vi "Lab Panel V4.83.vi"() -> ()   [LabVIEW 2013] (continued)
                        n580 = case shown="\"CYCLE TEST\"" w902 {
                          tunnel: w900 -> [_ _ w909]
                          tunnel: w899 -> [w907 w908 _]
                          tunnel: [w907 w908 w909] -> w898
                          frame "CHART TEST", Default {
                          }
                          frame "CYCLE TEST" {
                          }
                          frame "T-RISE TEST" {
                          }
                        }
                        n581 = local read "TDMS LAB02-2"() -> (w906:refnum<k34>)
                        n582 = Build Array("STOPPED") -> (w903:string[])
                        n583 = Build Array(w898) -> (w897:dbl[])
                        n584 = TDMS Write(0:w906, 5:"TEST RESULT", 7:w903, 9:w897) -> (4:w895:refnum<k34>, 15:w896:errorcluster)  [unwired: 2 in, 2 out]
                        n585 = TDMS Close(8:w896, 11:w895) -> (0:w894:errorcluster)  [unwired: 1 out]
                      }
                      frame #1 {
                        n586 = local read "DISP LAB02-2"() -> (w913:T4)
                        n587 = stacked-sequence {
                          tunnel: "LAB02-2" -> [w915 w917]
                          frame #0 {
                            n588 = call "sub vi - defrag tdms v1.vi"("panel id"=w915) -> ("error out"=w914:errorcluster)  [unwired: 10 in]
                            n589 = local write "data file error"(w914) -> ()
                          }
                          frame #1 {
                            n590 = call "Save data file to network drive v1.vi"("panel id"=w917) -> ("network file save error"=w916:errorcluster)  [unwired: 9 in, 1 out]
                            n591 = local write "RESULT LAB02-2"(FALSE) -> ()
                            n592 = local write "data file error"(w916) -> ()
                          }
                        }
                        n593 = Bundle(cluster=w913, "STATUS"="STOP") -> (w911:T4)  [unwired: 2 in]
                        n594 = local write "DISP LAB02-2"(w911) -> ()
                      }
                    }
                  }
                  frame True {
                    # "start new test and create test file"
                    n595 = stacked-sequence {
                      seq-local: [w925 _ _ _ _] -> [_ w950 _ _ _]
                      tunnel: w924 -> [w930 _ _ _ _]
                      tunnel: w923 -> [w927 _ _ _ _]
                      tunnel: w922 -> [w940 _ _ _ _]
                      tunnel: w921 -> [w933 _ _ _ _]
                      tunnel: w920 -> [w928 _ _ _ _]
                      tunnel: [_ w944 _ _ _] -> w919
                      frame #0 {
                        w926 = "\\"
                        n596 = local read "SET LAB02-2"() -> (w935:T5)
                        n597 = case shown="\"CYCLE TEST\"" w940 {
                          tunnel: ["L02-2-CHART TEST-" "L02-2-CYCLE TEST-" "L02-2-T-RISE TEST-"] -> w936
                          frame "CHART TEST", Default {
                          }
                          frame "CYCLE TEST" {
                          }
                          frame "T-RISE TEST" {
                          }
                        }
                        n598 = Unbundle(w935) -> ("DESCRIPTION"=w934:string)  [unwired: 4 out]
                        n599 = Concatenate Strings(w930, "\\", w928, w926, w927, w926) -> (w937:string)
                        n600 = String To Path(string=w937) -> (path=w939:path)
                        n601 = Concatenate Strings(w937, w936, w934, "-", w933, ".tdms") -> (w925:string)
                        n602 = Create Folder(path (use dialog)=w939) -> (error out=w938:errorcluster)  [unwired: 2 in, 2 out]
                        n603 = global write "Global 1.vi" "LAB02-2 FILE"(w925) -> ()
                        n604 = call <vilib>:"Clear Errors.vi"("error in (no error)"=w938) -> ()  [unwired: 6 in, 1 out]
                      }
                      frame #1 {
                        n605 = String To Path(string=w950) -> (path=w945:path)
                        n606 = TDMS Open(5:FALSE, 6:FALSE, 10:T18."create or replace" ("operation (0:open)"), 11:w945) -> (0:w944:errorcluster, 3:→"TDMS LAB02-2":refnum<k34>)  [unwired: 3 in]
                      }
                      frame #2 {
                        n607 = local read "SET LAB02-2"() -> (w956:T5)
                        n608 = local read "TDMS LAB02-2"() -> (w967:refnum<k34>)
                        n609 = Build Array("Testers Name", "Description", "Set Test Cycles", "T-Rise minutes", "T-Rise Deg C") -> (w957:string[])
                        n610 = Unbundle(w956) -> ("NAME"=w955:string, "DESCRIPTION"=w954:string, "CYCLES"=w953:dbl, "T-RISE mins"=w952:dbl, "T-RISE deg C"=w951:dbl)
                        n611 = Number To Decimal String(number=w953) -> (decimal integer string=w966:string)  [unwired: 1 in]
                        n612 = Number To Decimal String(number=w952) -> (decimal integer string=w965:string)  [unwired: 1 in]
                        n613 = Number To Decimal String(number=w951) -> (decimal integer string=w964:string)  [unwired: 1 in]
                        n614 = Build Array(w955, w954, w966, w965, w964) -> (w963:string[])
                        n615 = TDMS Set Properties(5:w963, 7:w957, 11:w967) -> ()  [unwired: 3 in, 4 out]
                      }
                      frame #3 {
                        w969 = 0.0
                        n616 = local read "DISP LAB02-2"() -> (w971:T4)
                        n617 = Bundle(cluster=w971, "CYCLE"=w969, "MINS"=w969, "STATUS"="RUN") -> (w970:T4)
                        n618 = local write "DISP LAB02-2"(w970) -> ()
                      }
                      frame #4 {
                        n619 = local read "SIG LAB02-2"() -> (w974:T2)
                        n620 = local read "TEMP START LAB02-2"() -> (w976:cluster{"TL":dbl, "TN":dbl})
                        n621 = Unbundle(w974) -> ("Tmp Live"=w973:dbl, "Tmp Neut"=w972:dbl)  [unwired: 3 out]
                        n622 = Bundle(cluster=w976, "TL"=w973, "TN"=w972) -> (w975:cluster{"TL":dbl, "TN":dbl})
                        n623 = local write "TEMP START LAB02-2"(w975) -> ()
                      }
                    }
                  }
                }
              }
              event "RUN LAB03-1": Value Change {
                n624 = event-data() -> ("NewVal"=w977:bool)  [unwired: 1 in, 5 out]
                n625 = local write "run lab03-1"(w977) -> ()
                n626 = case shown="True" w977 {
                  tunnel: w983 -> [_ w1016]
                  tunnel: w982 -> [_ w1015]
                  tunnel: w980 -> [w985 w1014]
                  tunnel: w981 -> [_ w1013]
                  tunnel: w979 -> [_ w1012]
                  tunnel: [w984 w1011] -> w978
                  frame False {
                    # "stop test"
                    n627 = stacked-sequence {
                      tunnel: w985 -> [w994 _]
                      tunnel: [w986 _] -> w984
                      frame #0 {
                        n628 = local read "DISP LAB03-1"() -> (w993:T4)
                        n629 = Unbundle(w993) -> ("CYCLE"=w991:dbl, "MINS"=w992:dbl)  [unwired: 1 out]
                        n630 = case shown="\"CYCLE TEST\"" w994 {
                          tunnel: w992 -> [_ _ w1001]
                          tunnel: w991 -> [w999 w1000 _]
                          tunnel: [w999 w1000 w1001] -> w990
                          frame "CHART TEST", Default {
                          }
                          frame "CYCLE TEST" {
                          }
                          frame "T-RISE TEST" {
                          }
                        }
                        n631 = local read "TDMS LAB03-1"() -> (w998:refnum<k34>)
                        n632 = Build Array("STOPPED") -> (w995:string[])
                        n633 = Build Array(w990) -> (w989:dbl[])
                        n634 = TDMS Write(0:w998, 5:"TEST RESULT", 7:w995, 9:w989) -> (4:w987:refnum<k34>, 15:w988:errorcluster)  [unwired: 2 in, 2 out]
                        n635 = TDMS Close(8:w988, 11:w987) -> (0:w986:errorcluster)  [unwired: 1 out]
                      }
                      frame #1 {
                        n636 = local read "DISP LAB03-1"() -> (w1005:T4)
                        n637 = stacked-sequence {
                          tunnel: "LAB03-1" -> [w1007 w1009]
                          frame #0 {
                            n638 = call "sub vi - defrag tdms v1.vi"("panel id"=w1007) -> ("error out"=w1006:errorcluster)  [unwired: 10 in]
                            n639 = local write "data file error"(w1006) -> ()
                          }
                          frame #1 {
                            n640 = call "Save data file to network drive v1.vi"("panel id"=w1009) -> ("network file save error"=w1008:errorcluster)  [unwired: 9 in, 1 out]
                            n641 = local write "RESULT LAB03-1"(FALSE) -> ()
                            n642 = local write "data file error"(w1008) -> ()
                          }
                        }
                        n643 = Bundle(cluster=w1005, "STATUS"="STOP") -> (w1003:T4)  [unwired: 2 in]
                        n644 = local write "DISP LAB03-1"(w1003) -> ()
                      }
                    }
                  }
                  frame True {
                    # "start new test and create test file"
                    n645 = stacked-sequence {
                      seq-local: [w1017 _ _ _ _] -> [_ w1042 _ _ _]
                      tunnel: w1016 -> [w1022 _ _ _ _]
                      tunnel: w1015 -> [w1019 _ _ _ _]
                      tunnel: w1014 -> [w1032 _ _ _ _]
                      tunnel: w1013 -> [w1025 _ _ _ _]
                      tunnel: w1012 -> [w1020 _ _ _ _]
                      tunnel: [_ w1036 _ _ _] -> w1011
                      frame #0 {
                        w1018 = "\\"
                        n646 = local read "SET LAB03-1"() -> (w1027:T5)
                        n647 = case shown="\"T-RISE TEST\"" w1032 {
                          tunnel: ["L03-1-CHART TEST-" "L03-1-CYCLE TEST-" "L03-1-T-RISE TEST-"] -> w1028
                          frame "CHART TEST", Default {
                          }
                          frame "CYCLE TEST" {
                          }
                          frame "T-RISE TEST" {
                          }
                        }
                        n648 = Unbundle(w1027) -> ("DESCRIPTION"=w1026:string)  [unwired: 4 out]
                        n649 = Concatenate Strings(w1022, "\\", w1020, w1018, w1019, w1018) -> (w1029:string)
                        n650 = String To Path(string=w1029) -> (path=w1031:path)
                        n651 = Concatenate Strings(w1029, w1028, w1026, "-", w1025, ".tdms") -> (w1017:string)
                        n652 = Create Folder(path (use dialog)=w1031) -> (error out=w1030:errorcluster)  [unwired: 2 in, 2 out]
                        n653 = global write "Global 1.vi" "LAB03-1 FILE"(w1017) -> ()
                        n654 = call <vilib>:"Clear Errors.vi"("error in (no error)"=w1030) -> ()  [unwired: 6 in, 1 out]
                      }
                      frame #1 {
                        n655 = String To Path(string=w1042) -> (path=w1037:path)
                        n656 = TDMS Open(5:FALSE, 6:FALSE, 10:T18."create or replace" ("operation (0:open)"), 11:w1037) -> (0:w1036:errorcluster, 3:→"TDMS LAB03-1":refnum<k34>)  [unwired: 3 in]
                      }
                      frame #2 {
                        n657 = local read "SET LAB03-1"() -> (w1048:T5)
                        n658 = local read "TDMS LAB03-1"() -> (w1059:refnum<k34>)
                        n659 = Build Array("Testers Name", "Description", "Set Test Cycles", "T-Rise minutes", "T-Rise Deg C") -> (w1049:string[])
                        n660 = Unbundle(w1048) -> ("NAME"=w1047:string, "DESCRIPTION"=w1046:string, "CYCLES"=w1045:dbl, "T-RISE mins"=w1044:dbl, "T-RISE deg C"=w1043:dbl)
                        n661 = Number To Decimal String(number=w1045) -> (decimal integer string=w1058:string)  [unwired: 1 in]
                        n662 = Number To Decimal String(number=w1044) -> (decimal integer string=w1057:string)  [unwired: 1 in]
                        n663 = Number To Decimal String(number=w1043) -> (decimal integer string=w1056:string)  [unwired: 1 in]
                        n664 = Build Array(w1047, w1046, w1058, w1057, w1056) -> (w1055:string[])
                        n665 = TDMS Set Properties(5:w1055, 7:w1049, 11:w1059) -> ()  [unwired: 3 in, 4 out]
                      }
                      frame #3 {
                        w1061 = 0.0
                        n666 = local read "DISP LAB03-1"() -> (w1063:T4)
                        n667 = Bundle(cluster=w1063, "CYCLE"=w1061, "MINS"=w1061, "STATUS"="RUN") -> (w1062:T4)
                        n668 = local write "DISP LAB03-1"(w1062) -> ()
                      }
                      frame #4 {
                        n669 = local read "SIG LAB03-1"() -> (w1066:T2)
                        n670 = local read "TEMP START LAB03-1"() -> (w1068:cluster{"TL":dbl, "TN":dbl})
                        n671 = Unbundle(w1066) -> ("Tmp Live"=w1065:dbl, "Tmp Neut"=w1064:dbl)  [unwired: 3 out]
                        n672 = Bundle(cluster=w1068, "TL"=w1065, "TN"=w1064) -> (w1067:cluster{"TL":dbl, "TN":dbl})
                        n673 = local write "TEMP START LAB03-1"(w1067) -> ()
                      }
                    }
                  }
                }
              }
              event "RUN LAB03-2": Value Change {
                n674 = event-data() -> ("NewVal"=w1069:bool)  [unwired: 1 in, 5 out]
                n675 = local write "run lab03-2"(w1069) -> ()
                n676 = case shown="True" w1069 {
                  tunnel: w1075 -> [_ w1108]
                  tunnel: w1074 -> [_ w1107]
                  tunnel: w1072 -> [w1077 w1106]
                  tunnel: w1073 -> [_ w1105]
                  tunnel: w1071 -> [_ w1104]
                  tunnel: [w1076 w1103] -> w1070
                  frame False {
                    # "stop test"
                    n677 = stacked-sequence {
                      tunnel: w1077 -> [w1086 _]
                      tunnel: [w1078 _] -> w1076
                      frame #0 {
                        n678 = local read "DISP LAB03-2"() -> (w1085:T4)
                        n679 = Unbundle(w1085) -> ("CYCLE"=w1083:dbl, "MINS"=w1084:dbl)  [unwired: 1 out]
                        n680 = case shown="\"CYCLE TEST\"" w1086 {
                          tunnel: w1084 -> [_ _ w1093]
                          tunnel: w1083 -> [w1091 w1092 _]
                          tunnel: [w1091 w1092 w1093] -> w1082
                          frame "CHART TEST", Default {
                          }
                          frame "CYCLE TEST" {
                          }
                          frame "T-RISE TEST" {
                          }
                        }
                        n681 = local read "TDMS LAB03-2"() -> (w1090:refnum<k34>)
                        n682 = Build Array("STOPPED") -> (w1087:string[])
                        n683 = Build Array(w1082) -> (w1081:dbl[])
                        n684 = TDMS Write(0:w1090, 5:"TEST RESULT", 7:w1087, 9:w1081) -> (4:w1079:refnum<k34>, 15:w1080:errorcluster)  [unwired: 2 in, 2 out]
                        n685 = TDMS Close(8:w1080, 11:w1079) -> (0:w1078:errorcluster)  [unwired: 1 out]
                      }
                      frame #1 {
                        n686 = local read "DISP LAB03-2"() -> (w1097:T4)
                        n687 = stacked-sequence {
                          tunnel: "LAB03-2" -> [w1099 w1101]
                          frame #0 {
                            n688 = call "sub vi - defrag tdms v1.vi"("panel id"=w1099) -> ("error out"=w1098:errorcluster)  [unwired: 10 in]
                            n689 = local write "data file error"(w1098) -> ()
                          }
                          frame #1 {
                            n690 = call "Save data file to network drive v1.vi"("panel id"=w1101) -> ("network file save error"=w1100:errorcluster)  [unwired: 9 in, 1 out]
                            n691 = local write "RESULT LAB03-2"(FALSE) -> ()
                            n692 = local write "data file error"(w1100) -> ()
                          }
                        }
                        n693 = Bundle(cluster=w1097, "STATUS"="STOP") -> (w1095:T4)  [unwired: 2 in]
                        n694 = local write "DISP LAB03-2"(w1095) -> ()
                      }
                    }
                  }
                  frame True {
                    # "start new test and create test file"
                    n695 = stacked-sequence {
                      seq-local: [w1109 _ _ _ _] -> [_ w1134 _ _ _]
                      tunnel: w1108 -> [w1114 _ _ _ _]
                      tunnel: w1107 -> [w1111 _ _ _ _]
                      tunnel: w1106 -> [w1124 _ _ _ _]
                      tunnel: w1105 -> [w1117 _ _ _ _]
                      tunnel: w1104 -> [w1112 _ _ _ _]
                      tunnel: [_ w1128 _ _ _] -> w1103
                      frame #0 {
                        w1110 = "\\"
                        n696 = local read "SET LAB03-2"() -> (w1119:T5)
                        n697 = case shown="\"T-RISE TEST\"" w1124 {
                          tunnel: ["L03-2-CHART TEST-" "L03-2-CYCLE TEST-" "L03-2-T-RISE TEST-"] -> w1120
                          frame "CHART TEST", Default {
                          }
                          frame "CYCLE TEST" {
                          }
                          frame "T-RISE TEST" {
                          }
                        }
                        n698 = Unbundle(w1119) -> ("DESCRIPTION"=w1118:string)  [unwired: 4 out]
                        n699 = Concatenate Strings(w1114, "\\", w1112, w1110, w1111, w1110) -> (w1121:string)
                        n700 = String To Path(string=w1121) -> (path=w1123:path)
                        n701 = Concatenate Strings(w1121, w1120, w1118, "-", w1117, ".tdms") -> (w1109:string)
                        n702 = Create Folder(path (use dialog)=w1123) -> (error out=w1122:errorcluster)  [unwired: 2 in, 2 out]
                        n703 = global write "Global 1.vi" "LAB03-2 FILE"(w1109) -> ()
                        n704 = call <vilib>:"Clear Errors.vi"("error in (no error)"=w1122) -> ()  [unwired: 6 in, 1 out]
                      }
                      frame #1 {
                        n705 = String To Path(string=w1134) -> (path=w1129:path)
                        n706 = TDMS Open(5:FALSE, 6:FALSE, 10:T18."create or replace" ("operation (0:open)"), 11:w1129) -> (0:w1128:errorcluster, 3:→"TDMS LAB03-2":refnum<k34>)  [unwired: 3 in]
                      }
                      frame #2 {
                        n707 = local read "SET LAB03-2"() -> (w1140:T5)
                        n708 = local read "TDMS LAB03-2"() -> (w1151:refnum<k34>)
                        n709 = Build Array("Testers Name", "Description", "Set Test Cycles", "T-Rise minutes", "T-Rise Deg C") -> (w1141:string[])
                        n710 = Unbundle(w1140) -> ("NAME"=w1139:string, "DESCRIPTION"=w1138:string, "CYCLES"=w1137:dbl, "T-RISE mins"=w1136:dbl, "T-RISE deg C"=w1135:dbl)
                        n711 = Number To Decimal String(number=w1137) -> (decimal integer string=w1150:string)  [unwired: 1 in]
                        n712 = Number To Decimal String(number=w1136) -> (decimal integer string=w1149:string)  [unwired: 1 in]
                        n713 = Number To Decimal String(number=w1135) -> (decimal integer string=w1148:string)  [unwired: 1 in]
                        n714 = Build Array(w1139, w1138, w1150, w1149, w1148) -> (w1147:string[])
                        n715 = TDMS Set Properties(5:w1147, 7:w1141, 11:w1151) -> ()  [unwired: 3 in, 4 out]
                      }
                      frame #3 {
                        w1153 = 0.0
                        n716 = local read "DISP LAB03-2"() -> (w1155:T4)
                        n717 = Bundle(cluster=w1155, "CYCLE"=w1153, "MINS"=w1153, "STATUS"="RUN") -> (w1154:T4)
                        n718 = local write "DISP LAB03-2"(w1154) -> ()
                      }
                      frame #4 {
                        n719 = local read "SIG LAB03-2"() -> (w1158:T2)
                        n720 = local read "TEMP START LAB03-2"() -> (w1160:cluster{"TL":dbl, "TN":dbl})
                        n721 = Unbundle(w1158) -> ("Tmp Live"=w1157:dbl, "Tmp Neut"=w1156:dbl)  [unwired: 3 out]
                        n722 = Bundle(cluster=w1160, "TL"=w1157, "TN"=w1156) -> (w1159:cluster{"TL":dbl, "TN":dbl})
                        n723 = local write "TEMP START LAB03-2"(w1159) -> ()
                      }
                    }
                  }
                }
              }
              event "RUN LAB04-1": Value Change {
                n724 = event-data() -> ("NewVal"=w1161:bool)  [unwired: 1 in, 5 out]
                n725 = local write "run lab04-1"(w1161) -> ()
                n726 = case shown="True" w1161 {
                  tunnel: w1167 -> [_ w1200]
                  tunnel: w1166 -> [_ w1199]
                  tunnel: w1164 -> [w1169 w1198]
                  tunnel: w1165 -> [_ w1197]
                  tunnel: w1163 -> [_ w1196]
                  tunnel: [w1168 w1195] -> w1162
                  frame False {
                    # "stop test"
                    n727 = stacked-sequence {
                      tunnel: w1169 -> [w1178 _]
                      tunnel: [w1170 _] -> w1168
                      frame #0 {
                        n728 = local read "DISP LAB04-1"() -> (w1177:T4)
                        n729 = Unbundle(w1177) -> ("CYCLE"=w1175:dbl, "MINS"=w1176:dbl)  [unwired: 1 out]
                        n730 = case shown="\"CYCLE TEST\"" w1178 {
                          tunnel: w1176 -> [_ _ w1185]
                          tunnel: w1175 -> [w1183 w1184 _]
                          tunnel: [w1183 w1184 w1185] -> w1174
                          frame "CHART TEST", Default {
                          }
                          frame "CYCLE TEST" {
                          }
                          frame "T-RISE TEST" {
                          }
                        }
                        n731 = local read "TDMS LAB04-1"() -> (w1182:refnum<k34>)
                        n732 = Build Array("STOPPED") -> (w1179:string[])
                        n733 = Build Array(w1174) -> (w1173:dbl[])
                        n734 = TDMS Write(0:w1182, 5:"TEST RESULT", 7:w1179, 9:w1173) -> (4:w1171:refnum<k34>, 15:w1172:errorcluster)  [unwired: 2 in, 2 out]
                        n735 = TDMS Close(8:w1172, 11:w1171) -> (0:w1170:errorcluster)  [unwired: 1 out]
                      }
                      frame #1 {
                        n736 = local read "DISP LAB04-1"() -> (w1189:T4)
                        n737 = stacked-sequence {
                          tunnel: "LAB04-1" -> [w1191 w1193]
                          frame #0 {
                            n738 = call "sub vi - defrag tdms v1.vi"("panel id"=w1191) -> ("error out"=w1190:errorcluster)  [unwired: 10 in]
                            n739 = local write "data file error"(w1190) -> ()
                          }
                          frame #1 {
                            n740 = call "Save data file to network drive v1.vi"("panel id"=w1193) -> ("network file save error"=w1192:errorcluster)  [unwired: 9 in, 1 out]
                            n741 = local write "RESULT LAB04-1"(FALSE) -> ()
                            n742 = local write "data file error"(w1192) -> ()
                          }
                        }
                        n743 = Bundle(cluster=w1189, "STATUS"="STOP") -> (w1187:T4)  [unwired: 2 in]
                        n744 = local write "DISP LAB04-1"(w1187) -> ()
                      }
                    }
                  }
                  frame True {
                    # "start new test and create test file"
                    n745 = stacked-sequence {
                      seq-local: [w1201 _ _ _ _] -> [_ w1226 _ _ _]
                      tunnel: w1200 -> [w1206 _ _ _ _]
                      tunnel: w1199 -> [w1202 _ _ _ _]
                      tunnel: w1198 -> [w1216 _ _ _ _]
                      tunnel: w1197 -> [w1209 _ _ _ _]
                      tunnel: w1196 -> [w1204 _ _ _ _]
                      tunnel: [_ w1220 _ _ _] -> w1195
                      frame #0 {
                        w1203 = "\\"
                        n746 = local read "SET LAB04-1"() -> (w1211:T5)
                        n747 = case shown="\"CYCLE TEST\"" w1216 {
                          tunnel: ["L04-1-CHART TEST-" "L04-1-CYCLE TEST-" "L04-1-T-RISE TEST-"] -> w1212
                          frame "CHART TEST", Default {
                          }
                          frame "CYCLE TEST" {
                          }
                          frame "T-RISE TEST" {
                          }
                        }
                        n748 = Unbundle(w1211) -> ("DESCRIPTION"=w1210:string)  [unwired: 4 out]
                        n749 = Concatenate Strings(w1206, "\\", w1204, w1203, w1202, w1203) -> (w1213:string)
                        n750 = String To Path(string=w1213) -> (path=w1215:path)
                        n751 = Concatenate Strings(w1213, w1212, w1210, "-", w1209, ".tdms") -> (w1201:string)
                        n752 = Create Folder(path (use dialog)=w1215) -> (error out=w1214:errorcluster)  [unwired: 2 in, 2 out]
                        n753 = global write "Global 1.vi" "LAB04-1 FILE"(w1201) -> ()
                        n754 = call <vilib>:"Clear Errors.vi"("error in (no error)"=w1214) -> ()  [unwired: 6 in, 1 out]
                      }
                      frame #1 {
                        n755 = String To Path(string=w1226) -> (path=w1221:path)
                        n756 = TDMS Open(5:FALSE, 6:FALSE, 10:T18."create or replace" ("operation (0:open)"), 11:w1221) -> (0:w1220:errorcluster, 3:→"TDMS LAB04-1":refnum<k34>)  [unwired: 3 in]
                      }
                      frame #2 {
                        n757 = local read "SET LAB04-1"() -> (w1232:T5)
                        n758 = local read "TDMS LAB04-1"() -> (w1243:refnum<k34>)
                        n759 = Build Array("Testers Name", "Description", "Set Test Cycles", "T-Rise minutes", "T-Rise Deg C") -> (w1233:string[])
                        n760 = Unbundle(w1232) -> ("NAME"=w1231:string, "DESCRIPTION"=w1230:string, "CYCLES"=w1229:dbl, "T-RISE mins"=w1228:dbl, "T-RISE deg C"=w1227:dbl)
                        n761 = Number To Decimal String(number=w1229) -> (decimal integer string=w1242:string)  [unwired: 1 in]
                        n762 = Number To Decimal String(number=w1228) -> (decimal integer string=w1241:string)  [unwired: 1 in]
                        n763 = Number To Decimal String(number=w1227) -> (decimal integer string=w1240:string)  [unwired: 1 in]
                        n764 = Build Array(w1231, w1230, w1242, w1241, w1240) -> (w1239:string[])
                        n765 = TDMS Set Properties(5:w1239, 7:w1233, 11:w1243) -> ()  [unwired: 3 in, 4 out]
                      }
                      frame #3 {
                        w1245 = 0.0
                        n766 = local read "DISP LAB04-1"() -> (w1247:T4)
                        n767 = Bundle(cluster=w1247, "CYCLE"=w1245, "MINS"=w1245, "STATUS"="RUN") -> (w1246:T4)
                        n768 = local write "DISP LAB04-1"(w1246) -> ()
                      }
                      frame #4 {
                        n769 = local read "SIG LAB04-1"() -> (w1250:T2)
                        n770 = local read "TEMP START LAB04-1"() -> (w1252:cluster{"TL":dbl, "TN":dbl})
                        n771 = Unbundle(w1250) -> ("Tmp Live"=w1249:dbl, "Tmp Neut"=w1248:dbl)  [unwired: 3 out]
                        n772 = Bundle(cluster=w1252, "TL"=w1249, "TN"=w1248) -> (w1251:cluster{"TL":dbl, "TN":dbl})
                        n773 = local write "TEMP START LAB04-1"(w1251) -> ()
                      }
                    }
                  }
                }
              }
              event "RUN LAB04-2": Value Change {
                n774 = event-data() -> ("NewVal"=w1253:bool)  [unwired: 1 in, 5 out]
                n775 = local write "run lab04-2"(w1253) -> ()
                n776 = case shown="True" w1253 {
                  tunnel: w1259 -> [_ w1292]
                  tunnel: w1258 -> [_ w1291]
                  tunnel: w1256 -> [w1261 w1290]
                  tunnel: w1257 -> [_ w1289]
                  tunnel: w1255 -> [_ w1288]
                  tunnel: [w1260 w1287] -> w1254
                  frame False {
                    # "stop test"
                    n777 = stacked-sequence {
                      tunnel: w1261 -> [w1270 _]
                      tunnel: [w1262 _] -> w1260
                      frame #0 {
                        n778 = local read "DISP LAB04-2"() -> (w1269:T4)
                        n779 = Unbundle(w1269) -> ("CYCLE"=w1267:dbl, "MINS"=w1268:dbl)  [unwired: 1 out]
                        n780 = case shown="\"CYCLE TEST\"" w1270 {
                          tunnel: w1268 -> [_ _ w1277]
                          tunnel: w1267 -> [w1275 w1276 _]
                          tunnel: [w1275 w1276 w1277] -> w1266
                          frame "CHART TEST", Default {
                          }
                          frame "CYCLE TEST" {
                          }
                          frame "T-RISE TEST" {
                          }
                        }
                        n781 = local read "TDMS LAB04-2"() -> (w1274:refnum<k34>)
                        n782 = Build Array("STOPPED") -> (w1271:string[])
                        n783 = Build Array(w1266) -> (w1265:dbl[])
                        n784 = TDMS Write(0:w1274, 5:"TEST RESULT", 7:w1271, 9:w1265) -> (4:w1263:refnum<k34>, 15:w1264:errorcluster)  [unwired: 2 in, 2 out]
                        n785 = TDMS Close(8:w1264, 11:w1263) -> (0:w1262:errorcluster)  [unwired: 1 out]
                      }
                      frame #1 {
                        n786 = local read "DISP LAB04-2"() -> (w1281:T4)
                        n787 = stacked-sequence {
                          tunnel: "LAB04-2" -> [w1283 w1285]
                          frame #0 {
                            n788 = call "sub vi - defrag tdms v1.vi"("panel id"=w1283) -> ("error out"=w1282:errorcluster)  [unwired: 10 in]
                            n789 = local write "data file error"(w1282) -> ()
                          }
                          frame #1 {
                            n790 = call "Save data file to network drive v1.vi"("panel id"=w1285) -> ("network file save error"=w1284:errorcluster)  [unwired: 9 in, 1 out]
                            n791 = local write "RESULT LAB04-2"(FALSE) -> ()
                            n792 = local write "data file error"(w1284) -> ()
                          }
                        }
                        n793 = Bundle(cluster=w1281, "STATUS"="STOP") -> (w1279:T4)  [unwired: 2 in]
                        n794 = local write "DISP LAB04-2"(w1279) -> ()
                      }
                    }
                  }
                  frame True {
                    # "start new test and create test file"
                    n795 = stacked-sequence {
                      seq-local: [w1293 _ _ _ _] -> [_ w1318 _ _ _]
                      tunnel: w1292 -> [w1298 _ _ _ _]
                      tunnel: w1291 -> [w1294 _ _ _ _]
                      tunnel: w1290 -> [w1308 _ _ _ _]
                      tunnel: w1289 -> [w1301 _ _ _ _]
                      tunnel: w1288 -> [w1296 _ _ _ _]
                      tunnel: [_ w1312 _ _ _] -> w1287
                      frame #0 {
                        w1295 = "\\"
                        n796 = local read "SET LAB04-2"() -> (w1303:T5)
                        n797 = case shown="\"CHART TEST\", Default" w1308 {
                          tunnel: ["L04-2-CHART TEST-" "L04-2-CYCLE TEST-" "L04-2-T-RISE TEST-"] -> w1304
                          frame "CHART TEST", Default {
                          }
                          frame "CYCLE TEST" {
                          }
                          frame "T-RISE TEST" {
                          }
                        }
                        n798 = Unbundle(w1303) -> ("DESCRIPTION"=w1302:string)  [unwired: 4 out]
                        n799 = Concatenate Strings(w1298, "\\", w1296, w1295, w1294, w1295) -> (w1305:string)
                        n800 = String To Path(string=w1305) -> (path=w1307:path)
                        n801 = Concatenate Strings(w1305, w1304, w1302, "-", w1301, ".tdms") -> (w1293:string)
                        n802 = Create Folder(path (use dialog)=w1307) -> (error out=w1306:errorcluster)  [unwired: 2 in, 2 out]
                        n803 = global write "Global 1.vi" "LAB04-2 FILE"(w1293) -> ()
                        n804 = call <vilib>:"Clear Errors.vi"("error in (no error)"=w1306) -> ()  [unwired: 6 in, 1 out]
                      }
                      frame #1 {
                        n805 = String To Path(string=w1318) -> (path=w1313:path)
                        n806 = TDMS Open(5:FALSE, 6:FALSE, 10:T18."create or replace" ("operation (0:open)"), 11:w1313) -> (0:w1312:errorcluster, 3:→"TDMS LAB04-2":refnum<k34>)  [unwired: 3 in]
                      }
                      frame #2 {
                        n807 = local read "SET LAB04-2"() -> (w1324:T5)
                        n808 = local read "TDMS LAB04-2"() -> (w1335:refnum<k34>)
                        n809 = Build Array("Testers Name", "Description", "Set Test Cycles", "T-Rise minutes", "T-Rise Deg C") -> (w1325:string[])
                        n810 = Unbundle(w1324) -> ("NAME"=w1323:string, "DESCRIPTION"=w1322:string, "CYCLES"=w1321:dbl, "T-RISE mins"=w1320:dbl, "T-RISE deg C"=w1319:dbl)
                        n811 = Number To Decimal String(number=w1321) -> (decimal integer string=w1334:string)  [unwired: 1 in]
                        n812 = Number To Decimal String(number=w1320) -> (decimal integer string=w1333:string)  [unwired: 1 in]
                        n813 = Number To Decimal String(number=w1319) -> (decimal integer string=w1332:string)  [unwired: 1 in]
                        n814 = Build Array(w1323, w1322, w1334, w1333, w1332) -> (w1331:string[])
                        n815 = TDMS Set Properties(5:w1331, 7:w1325, 11:w1335) -> ()  [unwired: 3 in, 4 out]
                      }
                      frame #3 {
                        w1337 = 0.0
                        n816 = local read "DISP LAB04-2"() -> (w1339:T4)
                        n817 = Bundle(cluster=w1339, "CYCLE"=w1337, "MINS"=w1337, "STATUS"="RUN") -> (w1338:T4)
                        n818 = local write "DISP LAB04-2"(w1338) -> ()
                      }
                      frame #4 {
                        n819 = local read "SIG LAB04-2"() -> (w1342:T2)
                        n820 = local read "TEMP START LAB04-2"() -> (w1344:cluster{"TL":dbl, "TN":dbl})
                        n821 = Unbundle(w1342) -> ("Tmp Live"=w1341:dbl, "Tmp Neut"=w1340:dbl)  [unwired: 3 out]
                        n822 = Bundle(cluster=w1344, "TL"=w1341, "TN"=w1340) -> (w1343:cluster{"TL":dbl, "TN":dbl})
                        n823 = local write "TEMP START LAB04-2"(w1343) -> ()
                      }
                    }
                  }
                }
              }
              event "RUN LAB05-1": Value Change {
                n824 = event-data() -> ("NewVal"=w1345:bool)  [unwired: 1 in, 5 out]
                n825 = local write "run lab05-1"(w1345) -> ()
                n826 = case shown="True" w1345 {
                  tunnel: w1351 -> [_ w1384]
                  tunnel: w1350 -> [_ w1383]
                  tunnel: w1348 -> [w1353 w1382]
                  tunnel: w1349 -> [_ w1381]
                  tunnel: w1347 -> [_ w1380]
                  tunnel: [w1352 w1379] -> w1346
                  frame False {
                    # "stop test"
                    n827 = stacked-sequence {
                      tunnel: w1353 -> [w1362 _]
                      tunnel: [w1354 _] -> w1352
                      frame #0 {
                        n828 = local read "DISP LAB05-1"() -> (w1361:T4)
                        n829 = Unbundle(w1361) -> ("CYCLE"=w1359:dbl, "MINS"=w1360:dbl)  [unwired: 1 out]
                        n830 = case shown="\"CYCLE TEST\"" w1362 {
                          tunnel: w1360 -> [_ _ w1369]
                          tunnel: w1359 -> [w1367 w1368 _]
                          tunnel: [w1367 w1368 w1369] -> w1358
                          frame "CHART TEST", Default {
                          }
                          frame "CYCLE TEST" {
                          }
                          frame "T-RISE TEST" {
                          }
                        }
                        n831 = local read "TDMS LAB05-1"() -> (w1366:refnum<k34>)
                        n832 = Build Array("STOPPED") -> (w1363:string[])
                        n833 = Build Array(w1358) -> (w1357:dbl[])
                        n834 = TDMS Write(0:w1366, 5:"TEST RESULT", 7:w1363, 9:w1357) -> (4:w1355:refnum<k34>, 15:w1356:errorcluster)  [unwired: 2 in, 2 out]
                        n835 = TDMS Close(8:w1356, 11:w1355) -> (0:w1354:errorcluster)  [unwired: 1 out]
                      }
                      frame #1 {
                        n836 = local read "DISP LAB05-1"() -> (w1373:T4)
                        n837 = stacked-sequence {
                          tunnel: "LAB05-1" -> [w1375 w1377]
                          frame #0 {
                            n838 = call "sub vi - defrag tdms v1.vi"("panel id"=w1375) -> ("error out"=w1374:errorcluster)  [unwired: 10 in]
                            n839 = local write "data file error"(w1374) -> ()
                          }
                          frame #1 {
                            n840 = call "Save data file to network drive v1.vi"("panel id"=w1377) -> ("network file save error"=w1376:errorcluster)  [unwired: 9 in, 1 out]
                            n841 = local write "RESULT LAB05-1"(FALSE) -> ()
                            n842 = local write "data file error"(w1376) -> ()
                          }
                        }
                        n843 = Bundle(cluster=w1373, "STATUS"="STOP") -> (w1371:T4)  [unwired: 2 in]
                        n844 = local write "DISP LAB05-1"(w1371) -> ()
                      }
                    }
                  }
                  frame True {
                    # "start new test and create test file"
                    n845 = stacked-sequence {
                      seq-local: [w1385 _ _ _ _] -> [_ w1410 _ _ _]
                      tunnel: w1384 -> [w1390 _ _ _ _]
                      tunnel: w1383 -> [w1386 _ _ _ _]
                      tunnel: w1382 -> [w1400 _ _ _ _]
                      tunnel: w1381 -> [w1393 _ _ _ _]
                      tunnel: w1380 -> [w1388 _ _ _ _]
                      tunnel: [_ w1404 _ _ _] -> w1379
                      frame #0 {
                        w1387 = "\\"
                        n846 = local read "SET LAB05-1"() -> (w1395:T5)
                        n847 = case shown="\"CYCLE TEST\"" w1400 {
                          tunnel: ["L05-1-CHART TEST-" "L05-1-CYCLE TEST-" "L05-1-T-RISE TEST-"] -> w1396
                          frame "CHART TEST", Default {
                          }
                          frame "CYCLE TEST" {
                          }
                          frame "T-RISE TEST" {
                          }
                        }
                        n848 = Unbundle(w1395) -> ("DESCRIPTION"=w1394:string)  [unwired: 4 out]
                        n849 = Concatenate Strings(w1390, "\\", w1388, w1387, w1386, w1387) -> (w1397:string)
                        n850 = String To Path(string=w1397) -> (path=w1399:path)
                        n851 = Concatenate Strings(w1397, w1396, w1394, "-", w1393, ".tdms") -> (w1385:string)
                        n852 = Create Folder(path (use dialog)=w1399) -> (error out=w1398:errorcluster)  [unwired: 2 in, 2 out]
                        n853 = global write "Global 1.vi" "LAB05-1 FILE"(w1385) -> ()
                        n854 = call <vilib>:"Clear Errors.vi"("error in (no error)"=w1398) -> ()  [unwired: 6 in, 1 out]
                      }
                      frame #1 {
                        n855 = String To Path(string=w1410) -> (path=w1405:path)
                        n856 = TDMS Open(5:FALSE, 6:FALSE, 10:T18."create or replace" ("operation (0:open)"), 11:w1405) -> (0:w1404:errorcluster, 3:→"TDMS LAB05-1":refnum<k34>)  [unwired: 3 in]
                      }
                      frame #2 {
                        n857 = local read "SET LAB05-1"() -> (w1416:T5)
                        n858 = local read "TDMS LAB05-1"() -> (w1427:refnum<k34>)
                        n859 = Build Array("Testers Name", "Description", "Set Test Cycles", "T-Rise minutes", "T-Rise Deg C") -> (w1417:string[])
                        n860 = Unbundle(w1416) -> ("NAME"=w1415:string, "DESCRIPTION"=w1414:string, "CYCLES"=w1413:dbl, "T-RISE mins"=w1412:dbl, "T-RISE deg C"=w1411:dbl)
                        n861 = Number To Decimal String(number=w1413) -> (decimal integer string=w1426:string)  [unwired: 1 in]
                        n862 = Number To Decimal String(number=w1412) -> (decimal integer string=w1425:string)  [unwired: 1 in]
                        n863 = Number To Decimal String(number=w1411) -> (decimal integer string=w1424:string)  [unwired: 1 in]
                        n864 = Build Array(w1415, w1414, w1426, w1425, w1424) -> (w1423:string[])
                        n865 = TDMS Set Properties(5:w1423, 7:w1417, 11:w1427) -> ()  [unwired: 3 in, 4 out]
                      }
                      frame #3 {
                        w1429 = 0.0
                        n866 = local read "DISP LAB05-1"() -> (w1431:T4)
                        n867 = Bundle(cluster=w1431, "CYCLE"=w1429, "MINS"=w1429, "STATUS"="RUN") -> (w1430:T4)
                        n868 = local write "DISP LAB05-1"(w1430) -> ()
                      }
                      frame #4 {
                        n869 = local read "SIG LAB05-1"() -> (w1434:T2)
                        n870 = local read "TEMP START LAB05-1"() -> (w1436:cluster{"TL":dbl, "TN":dbl})
                        n871 = Unbundle(w1434) -> ("Tmp Live"=w1433:dbl, "Tmp Neut"=w1432:dbl)  [unwired: 3 out]
                        n872 = Bundle(cluster=w1436, "TL"=w1433, "TN"=w1432) -> (w1435:cluster{"TL":dbl, "TN":dbl})
                        n873 = local write "TEMP START LAB05-1"(w1435) -> ()
                      }
                    }
                  }
                }
              }
              event "RUN LAB05-2": Value Change {
                n874 = event-data() -> ("NewVal"=w1437:bool)  [unwired: 1 in, 5 out]
                n875 = local write "run lab05-2"(w1437) -> ()
                n876 = case shown="True" w1437 {
                  tunnel: w1443 -> [_ w1476]
                  tunnel: w1442 -> [_ w1475]
                  tunnel: w1440 -> [w1445 w1474]
                  tunnel: w1441 -> [_ w1473]
                  tunnel: w1439 -> [_ w1472]
                  tunnel: [w1444 w1471] -> w1438
                  frame False {
                    # "stop test"
                    n877 = stacked-sequence {
                      tunnel: w1445 -> [w1454 _]
                      tunnel: [w1446 _] -> w1444
                      frame #0 {
                        n878 = local read "DISP LAB05-2"() -> (w1453:T4)
                        n879 = Unbundle(w1453) -> ("CYCLE"=w1451:dbl, "MINS"=w1452:dbl)  [unwired: 1 out]
                        n880 = case shown="\"CYCLE TEST\"" w1454 {
                          tunnel: w1452 -> [_ _ w1461]
                          tunnel: w1451 -> [w1459 w1460 _]
                          tunnel: [w1459 w1460 w1461] -> w1450
                          frame "CHART TEST", Default {
                          }
                          frame "CYCLE TEST" {
                          }
                          frame "T-RISE TEST" {
                          }
                        }
                        n881 = local read "TDMS LAB05-2"() -> (w1458:refnum<k34>)
                        n882 = Build Array("STOPPED") -> (w1455:string[])
                        n883 = Build Array(w1450) -> (w1449:dbl[])
                        n884 = TDMS Write(0:w1458, 5:"TEST RESULT", 7:w1455, 9:w1449) -> (4:w1447:refnum<k34>, 15:w1448:errorcluster)  [unwired: 2 in, 2 out]
                        n885 = TDMS Close(8:w1448, 11:w1447) -> (0:w1446:errorcluster)  [unwired: 1 out]
                      }
                      frame #1 {
                        n886 = local read "DISP LAB05-2"() -> (w1465:T4)
                        n887 = stacked-sequence {
                          tunnel: "LAB05-2" -> [w1467 w1469]
                          frame #0 {
                            n888 = call "sub vi - defrag tdms v1.vi"("panel id"=w1467) -> ("error out"=w1466:errorcluster)  [unwired: 10 in]
                            n889 = local write "data file error"(w1466) -> ()
                          }
                          frame #1 {
                            n890 = local write "RESULT LAB05-2"(FALSE) -> ()
                            n891 = call "Save data file to network drive v1.vi"("panel id"=w1469) -> ("network file save error"=w1468:errorcluster)  [unwired: 9 in, 1 out]
                            n892 = local write "data file error"(w1468) -> ()
                          }
                        }
                        n893 = Bundle(cluster=w1465, "STATUS"="STOP") -> (w1463:T4)  [unwired: 2 in]
                        n894 = local write "DISP LAB05-2"(w1463) -> ()
                      }
                    }
                  }
                  frame True {
                    # "start new test and create test file"
                    n895 = stacked-sequence {
                      seq-local: [w1477 _ _ _ _] -> [_ w1502 _ _ _]
                      tunnel: w1476 -> [w1482 _ _ _ _]
                      tunnel: w1475 -> [w1478 _ _ _ _]
                      tunnel: w1474 -> [w1492 _ _ _ _]
                      tunnel: w1473 -> [w1485 _ _ _ _]
                      tunnel: w1472 -> [w1480 _ _ _ _]
                      tunnel: [_ w1496 _ _ _] -> w1471
                      frame #0 {
                        w1479 = "\\"
                        n896 = local read "SET LAB05-2"() -> (w1487:T5)
                        n897 = case shown="\"CYCLE TEST\"" w1492 {
                          tunnel: ["L05-2-CHART TEST-" "L05-2-CYCLE TEST-" "L05-2-T-RISE TEST-"] -> w1488
                          frame "CHART TEST", Default {
                          }
                          frame "CYCLE TEST" {
                          }
                          frame "T-RISE TEST" {
                          }
                        }
                        n898 = Unbundle(w1487) -> ("DESCRIPTION"=w1486:string)  [unwired: 4 out]
                        n899 = Concatenate Strings(w1482, "\\", w1480, w1479, w1478, w1479) -> (w1489:string)
                        n900 = String To Path(string=w1489) -> (path=w1491:path)
                        n901 = Concatenate Strings(w1489, w1488, w1486, "-", w1485, ".tdms") -> (w1477:string)
                        n902 = Create Folder(path (use dialog)=w1491) -> (error out=w1490:errorcluster)  [unwired: 2 in, 2 out]
                        n903 = global write "Global 1.vi" "LAB05-2 FILE"(w1477) -> ()
                        n904 = call <vilib>:"Clear Errors.vi"("error in (no error)"=w1490) -> ()  [unwired: 6 in, 1 out]
                      }
                      frame #1 {
                        n905 = String To Path(string=w1502) -> (path=w1497:path)
                        n906 = TDMS Open(5:FALSE, 6:FALSE, 10:T18."create or replace" ("operation (0:open)"), 11:w1497) -> (0:w1496:errorcluster, 3:→"TDMS LAB05-2":refnum<k34>)  [unwired: 3 in]
                      }
                      frame #2 {
                        n907 = local read "SET LAB05-2"() -> (w1508:T5)
                        n908 = local read "TDMS LAB05-2"() -> (w1519:refnum<k34>)
                        n909 = Build Array("Testers Name", "Description", "Set Test Cycles", "T-Rise minutes", "T-Rise Deg C") -> (w1509:string[])
                        n910 = Unbundle(w1508) -> ("NAME"=w1507:string, "DESCRIPTION"=w1506:string, "CYCLES"=w1505:dbl, "T-RISE mins"=w1504:dbl, "T-RISE deg C"=w1503:dbl)
